vi "Close Execution Ref.vi"(8 "error in (no error)":errorcluster, 11 "teststand-api in":refnum<class "teststand-api.lvclass">) -> (0 "error out":errorcluster, 3 "teststand-api out":refnum<class "teststand-api.lvclass">)   [LabVIEW 2014, in "teststand-api.lvlib" / "teststand-api.lvclass"]
uses:
  teststand-api.lvclass
  teststand-api.lvclass/teststand-api.ctl
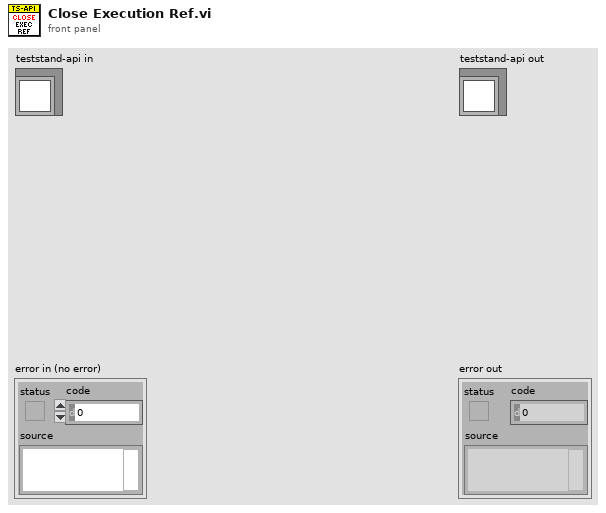
[diagram p1: front panel]
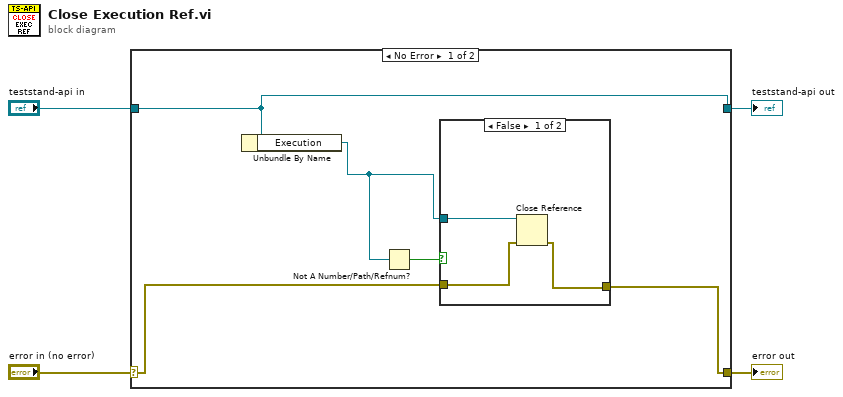
[diagram p0: block diagram]
diagram:
  n1 = case shown="No Error" "error in (no error)" {
    selector: "error in (no error)" -> [w6 w15]
    tunnel: [w5 w15] -> w3
    tunnel: [w9 w14] -> w1
    tunnel: "teststand-api in" -> [w9 w14]
    frame No Error {
      n2 = Unbundle By Name(w9) -> ("Execution"=w7:refnum<k7>)
      n3 = Not A Number/Path/Refnum?(number/path/refnum=w7) -> (NaN/Path/Refnum?=w8:bool)
      n4 = case shown="False" w8 {
        tunnel: w6 -> [w12 w13]
        tunnel: [w11 w13] -> w5
        tunnel: w7 -> [w10 _]
        frame False {
          n5 = Close Reference(reference=w10, error in (no error)=w12) -> (error out=w11:errorcluster)
        }
        frame True {
          # "ref is null, is not necessary to close it"
        }
      }
    }
    frame Error {
    }
  }
  "error out" <- w3
  "teststand-api out" <- w1
